vi "Manipulate XY Grid.vi"(8 "Deform Array":dbl[](array[numeric])=[1.0, 1.0, 1.0, 0.0, 0.0, 0.0, 0.0, 0.0, 0.0], 10 "XY Grid min In":dbl[](array[numeric])=[-4.0, 1.0], 11 "XY Quant. Fact. In":dbl[](array[numeric])=[1.0, 1.0]) -> (2 "XY Grid min Out":dbl[](array[numeric])=[-4.0, 1.0], 3 "XY Quant. Fact. Out":dbl[](array[numeric])=[1.0, 1.0])   [LabVIEW 2016]
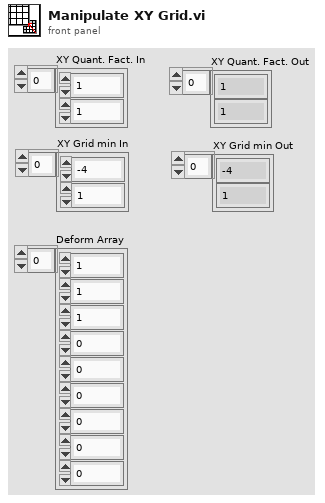
[diagram p1: front panel]
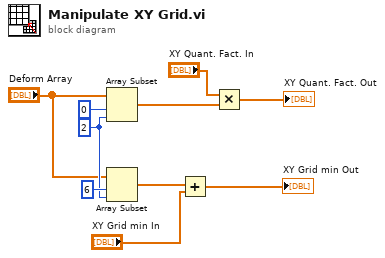
[diagram p0: block diagram]
diagram:
  w8 = 2 ("length")
  n1 = Array Subset(array="Deform Array", index=0, length=w8) -> (w7:dbl[])
  n2 = Array Subset(array="Deform Array", index=6, length=w8) -> (w5:dbl[])
  n3 = Add(x=w5, y="XY Grid min In") -> (x+y=→"XY Grid min Out":dbl[])
  n4 = Multiply(x="XY Quant. Fact. In", y=w7) -> (x*y=→"XY Quant. Fact. Out":dbl[])
